vi "Write code1.vi"(8 "error in (no error)":errorcluster, 10 "code1":dbl, 11 "Child in":refnum<class "Child.lvclass">) -> (0 "error out":errorcluster, 3 "Child out":refnum<class "Child.lvclass">)   [LabVIEW 2024, in "Child.lvclass"]
uses:
  Child.lvclass
  Child.lvclass/Child.ctl
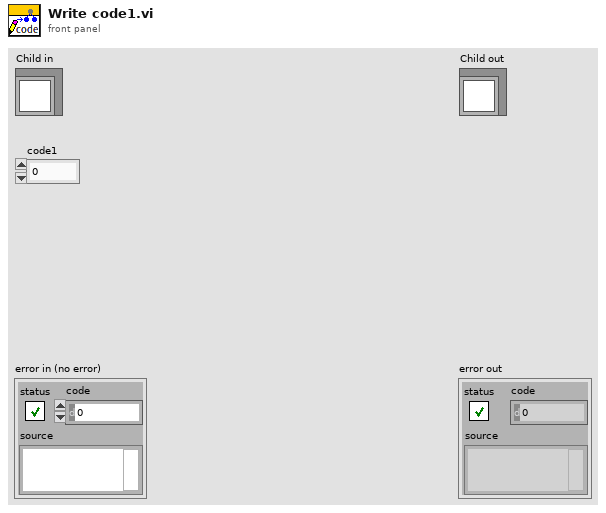
[diagram p1: front panel]
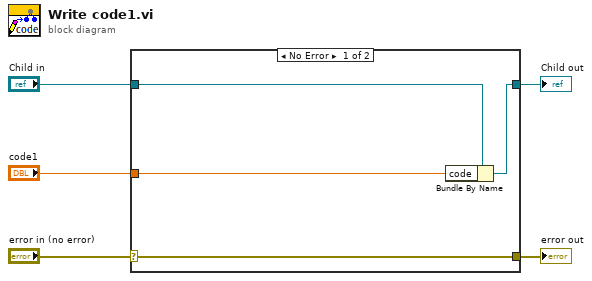
[diagram p0: block diagram]
diagram:
  n1 = case shown="No Error" "error in (no error)" {
    selector: "error in (no error)" -> [w9 w10]
    tunnel: [w9 w10] -> w4
    tunnel: [w7 w11] -> w2
    tunnel: "Child in" -> [w8 w11]
    tunnel: "code1" -> [w6 _]
    frame No Error {
      n2 = Bundle By Name(cluster=w8, "code"=w6) -> (w7:refnum<class "Child.lvclass">)
    }
    frame Error {
    }
  }
  "error out" <- w4
  "Child out" <- w2
